vi "ReadPressure.vi"(11 "Device Data":T1 {"IDS" format="%.0x"; "IDL" format="%.0x"; "IDM" format="%.0x"; "IDH" format="%.0x"}) -> (1 "Unit":string, 2 "Pressure":sgl, 3 "Function Output Comment":string, 4 "Message":string)   [LabVIEW 2019]
uses:
  Device Data.ctl
  164J027_AD/Brooks DLL 1.0.1.0 32bit/Brooks DLL 1.0.1.0 Release 10032016/S Protocol/BrooksDLL.dll
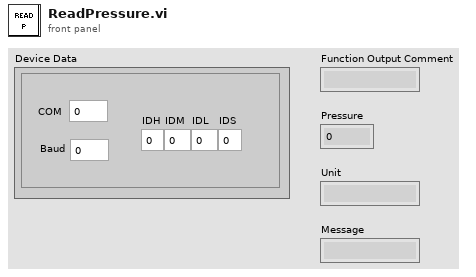
[diagram p1: front panel]
types:
  T1 = typedef "Device Data.ctl" = cluster{"COM":i32, "Baud":i32, "IDH":u8, "IDM":u8, "IDL":u8, "IDS":u8}
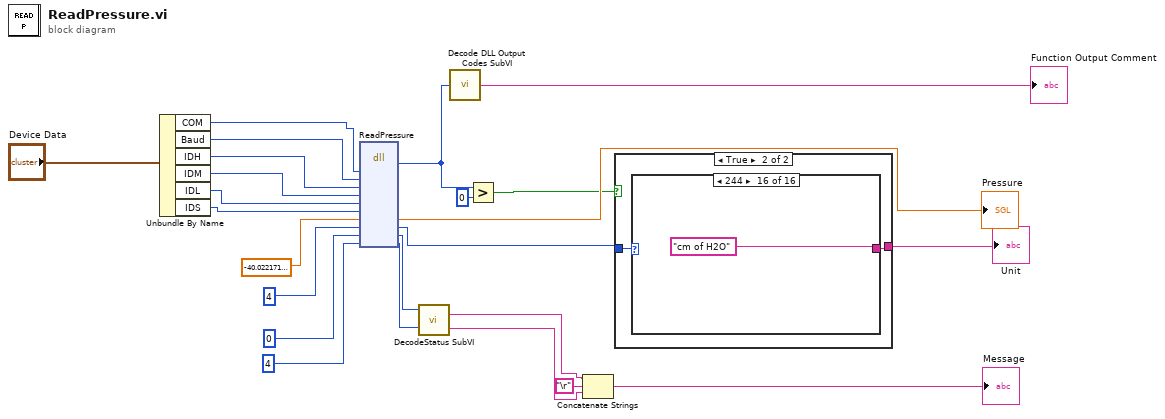
[diagram p0: block diagram]
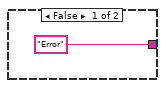
[diagram p2: hidden frame]
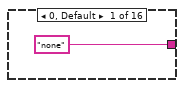
[diagram p3: hidden frame]
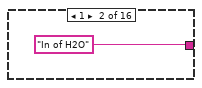
[diagram p4: hidden frame]
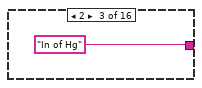
[diagram p5: hidden frame]
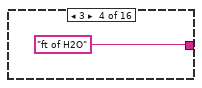
[diagram p6: hidden frame]
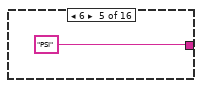
[diagram p7: hidden frame]
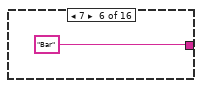
[diagram p8: hidden frame]
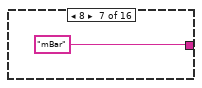
[diagram p9: hidden frame]
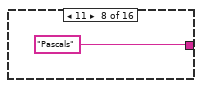
[diagram p10: hidden frame]
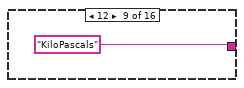
[diagram p11: hidden frame]
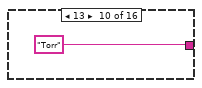
[diagram p12: hidden frame]
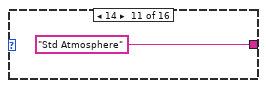
[diagram p13: hidden frame]
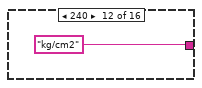
[diagram p14: hidden frame]
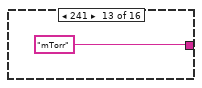
[diagram p15: hidden frame]
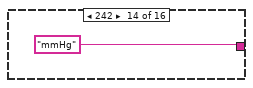
[diagram p16: hidden frame]
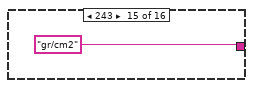
[diagram p17: hidden frame]
diagram:
  n1 = Unbundle By Name("Device Data") -> ("COM"=w19:i32, "Baud"=w20:i32, "IDH"=w24:u8, "IDM"=w23:u8, "IDL"=w22:u8, "IDS"=w21:u8)
  n2 = dll-call lib="G:/Developpement_de_Programmes/Programmes/Controle de pression/164J027_AD/Brooks DLL 1.0.1.0 32bit/Brooks DLL 1.0.1.0 Release 10032016/S Protocol/BrooksDLL.dll" fn="ReadPressure"("COM"=w19, "Baud"=w20, "IDH"=w24, "IDM"=w23, "IDL"=w22, "IDS"=w21, "Pressure"=sgl -40.02217, "PressureUnitCoce"=u8 4 ("Pressure Unit Code"), "S1"=u8 0 ("S1 2"), "S2"=u8 4 ("S2 2")) -> (w3:i32, "Pressure"=→"Pressure":sgl, "PressureUnitCoce"=w14:u8, "S1"=w4:u8, "S2"=w5:u8)  [unwired: 9 in, 2 out]
  n3 = call "DecodeStatus SubVI.vi"("S2"=w5, "S1"=w4) -> ("S2 String"=w12:string, "S1 String"=w11:string)
  n4 = call "Decode DLL Output Codes SubVI.vi"("Numeric"=w3) -> ("Function Output Comment"=→"Function Output Comment":string)
  n5 = Greater?(x=w3, y=0) -> (0:w1:bool)
  n6 = Concatenate Strings(w11, "\r" ("string"), w12) -> (→"Message":string)
  n7 = case shown="True" w1 {
    tunnel: w14 -> [_ w27]
    tunnel: ["Error" w26] -> w15
    frame False {
    }
    frame True {
      (unwired) ""
      n8 = case shown="244" w27 {
        tunnel: ["none" "In of H2O" "In of Hg" "ft of H2O" "PSI" "Bar" "mBar" "Pascals" "KiloPascals" "Torr" "Std Atmosphere" "kg/cm2" "mTorr" "mmHg" "gr/cm2" "cm of H2O"] -> w26
        frame 0, Default {
        }
        frame 1 {
        }
        frame 2 {
        }
        frame 3 {
        }
        frame 6 {
        }
        frame 7 {
        }
        frame 8 {
        }
        frame 11 {
        }
        frame 12 {
        }
        frame 13 {
        }
        frame 14 {
        }
        frame 240 {
        }
        frame 241 {
        }
        frame 242 {
        }
        frame 243 {
        }
        frame 244 {
        }
      }
    }
  }
  "Unit" <- w15
